vi "getType.vi"(8 "error in (no error)":errorcluster, 11 "Point in":refnum<class "Point.lvclass">) -> (0 "error out":errorcluster, 2 "type":enum16{"Point", "Loop", "Scan"}(ring), 3 "Point out":refnum<class "Point.lvclass">)   [LabVIEW 2009, in "Tools.lvlib" / "Sequencing.lvlib" / "Point.lvclass"]
uses:
  Point.lvclass
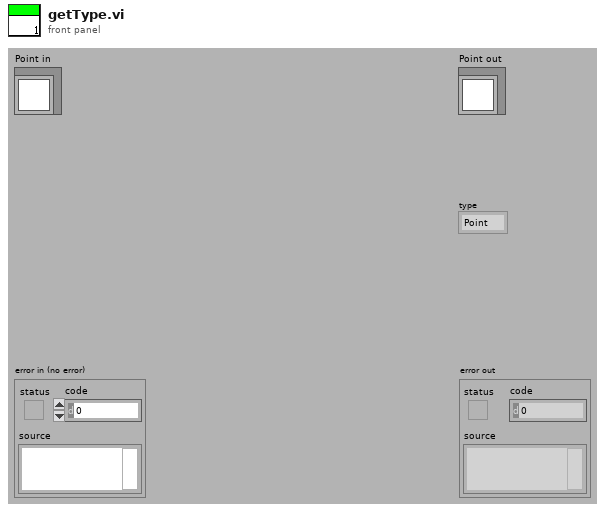
[diagram p1: front panel]
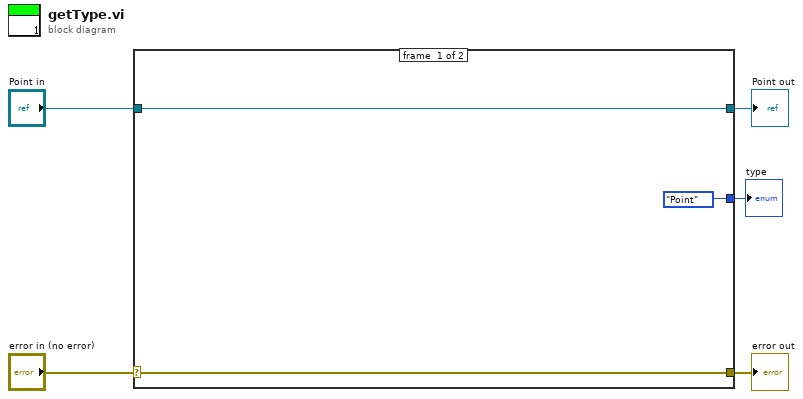
[diagram p0: block diagram]
diagram:
  n1 = case shown="No Error" "error in (no error)" {
    selector: "error in (no error)" -> [w7 w10]
    tunnel: [w7 w10] -> w4
    tunnel: [w8 w9] -> w2
    tunnel: "Point in" -> [w8 w9]
    tunnel: [enum16{"Point", "Loop", "Scan"}."Point" ("type") _] -> w1
    frame #0 {
    }
    frame #1 {
    }
  }
  "error out" <- w4
  "Point out" <- w2
  "type" <- w1
